vi "Emissor.vi"() -> ()   [LabVIEW 2012]
panel:
  out "error out":errorcluster
  in  "Numeric 2":dbl caption="Double"
  in  "Numeric":i64 caption="Inteiro"
  in  "String":string
  in  "Boolean":bool caption="TDD"
  in  "Ring":u16(ring) caption="Tipo de Dado" items=["String", "Inteiro", "Double"]
  # "Rodar Receptor.vi antes de rodar este VI."
  # "1- Escolher o tipo de Dado que será enviado;\n2- Preencher no controle escolhido;\n3- Rodar este VI."
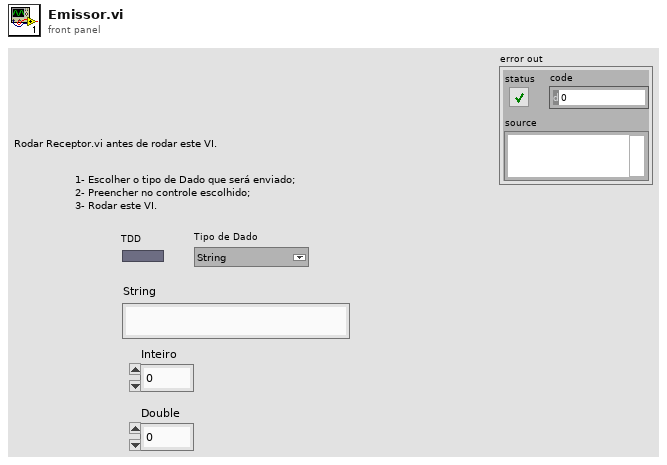
[diagram p1: front panel]
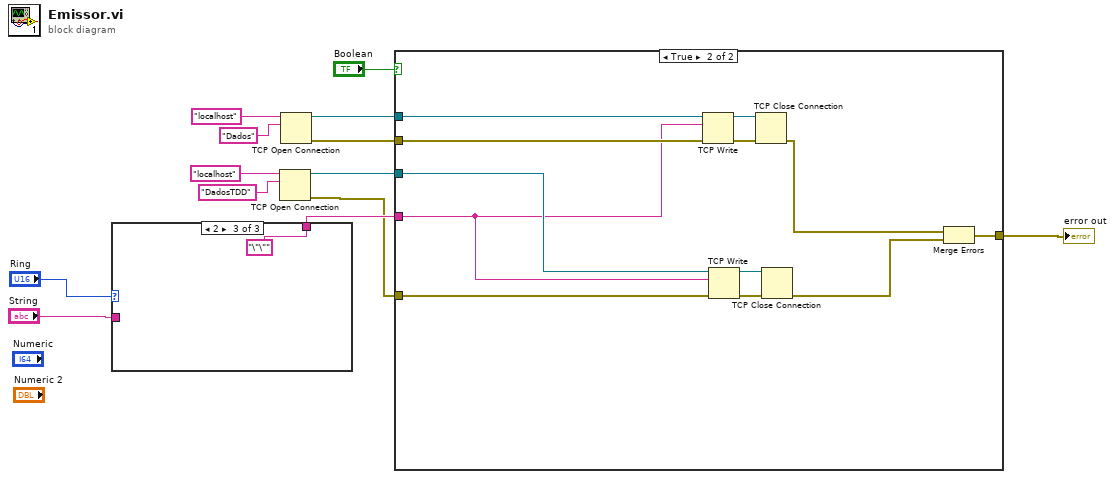
[diagram p0: block diagram]
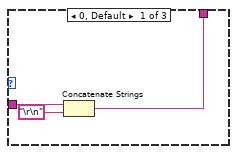
[diagram p2: hidden frame]
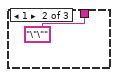
[diagram p3: hidden frame]
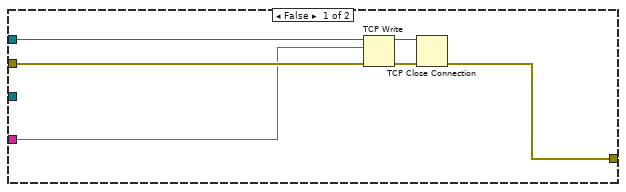
[diagram p4: hidden frame]
diagram:
  n1 = case shown="2" "Ring" {
    tunnel: "String" -> [w15 _ _]
    tunnel: [w14 "\"\"" "\"\""] -> w8
    frame 0, Default {
      n2 = Concatenate Strings(w15, "\r\n") -> (w14:string)
    }
    frame 1 {
    }
    frame 2 {
    }
  }
  n3 = TCP Open Connection(address="localhost", remote port or service name="DadosTDD" ("address")) -> (connection ID=w3:refnum<k5>, error out=w2:errorcluster)  [unwired: 1 in, 2 out]
  n4 = TCP Open Connection(address="localhost", remote port or service name="Dados" ("address")) -> (connection ID=w11:refnum<k5>, error out=w10:errorcluster)  [unwired: 1 in, 2 out]
  n5 = case shown="True" "Boolean" {
    tunnel: w11 -> [w24 w33]
    tunnel: w10 -> [w23 w34]
    tunnel: [w20 w26] -> w9
    tunnel: w8 -> [w19 w25]
    tunnel: w3 -> [_ w30]
    tunnel: w2 -> [_ w29]
    frame False {
      n6 = TCP Write(connection ID=w24, data in=w19, error in (no error)=w23) -> (connection ID out=w22:refnum<k5>, error out=w21:errorcluster)  [unwired: 2 out]
      n7 = TCP Close Connection(connection ID=w22, error in (no error)=w21) -> (error out=w20:errorcluster)  [unwired: 2 out]
    }
    frame True {
      n8 = TCP Write(connection ID=w33, data in=w25, error in (no error)=w34) -> (connection ID out=w36:refnum<k5>, error out=w35:errorcluster)  [unwired: 2 out]
      n9 = TCP Write(connection ID=w30, data in=w25, error in (no error)=w29) -> (connection ID out=w32:refnum<k5>, error out=w31:errorcluster)  [unwired: 2 out]
      n10 = TCP Close Connection(connection ID=w36, error in (no error)=w35) -> (error out=w28:errorcluster)  [unwired: 2 out]
      n11 = TCP Close Connection(connection ID=w32, error in (no error)=w31) -> (error out=w27:errorcluster)  [unwired: 2 out]
      n12 = Merge Errors(w28, w27) -> (w26:errorcluster)
    }
  }
  "error out" <- w9
